vi "Post-Build Action - PPL.vi"(5 "Files Generated by Build":path[](array[path]), 6 "Top Level/Always Included VIs":path[](array[path]), 7 "Destination Path":path, 8 "error in (no error)":errorcluster, 9 "Target Name":string, 10 "Build Specification Name":string, 11 "Project Path":path) -> (0 "error out":errorcluster)   [LabVIEW 2020]
doc: "<b>Post-Build Action</b>\nThis vi completes any post build actions needed for properly building the plugin."
uses:
  <vilib>/ADAS Record/Utilities/Config/Data Converter/Data Container and Version to JSON.vi
  <vilib>/ADAS Record/Utilities/ADAS Utilities.lvlib
  PE/ADAS PE Template.lvclass
  Controller/PE Controller.lvclass
panel:
  # "#via_ignore"
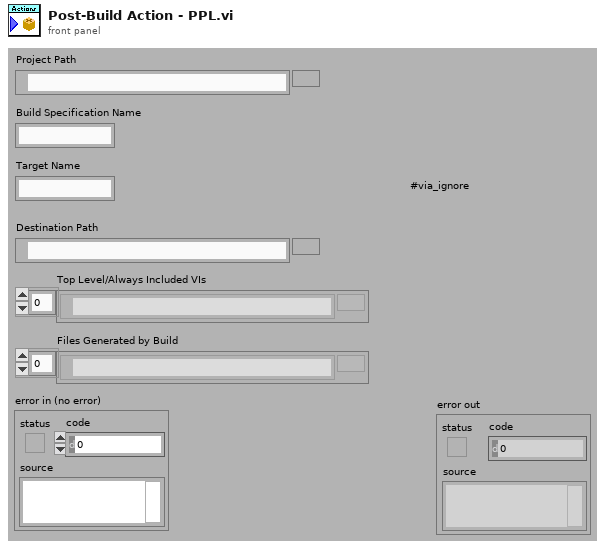
[diagram p1: front panel]
types:
  T1 = typedef "ADAS PE Template.lvlib/ADAS PE Template.lvclass/Configuration.ctl" = cluster{"Parameter1":string}
  T2 = typedef "ADAS Utilities.lvlib/Config Version.ctl" = cluster{"Major":u32, "Minor":u32, "Fix":u32, "Build":u32}
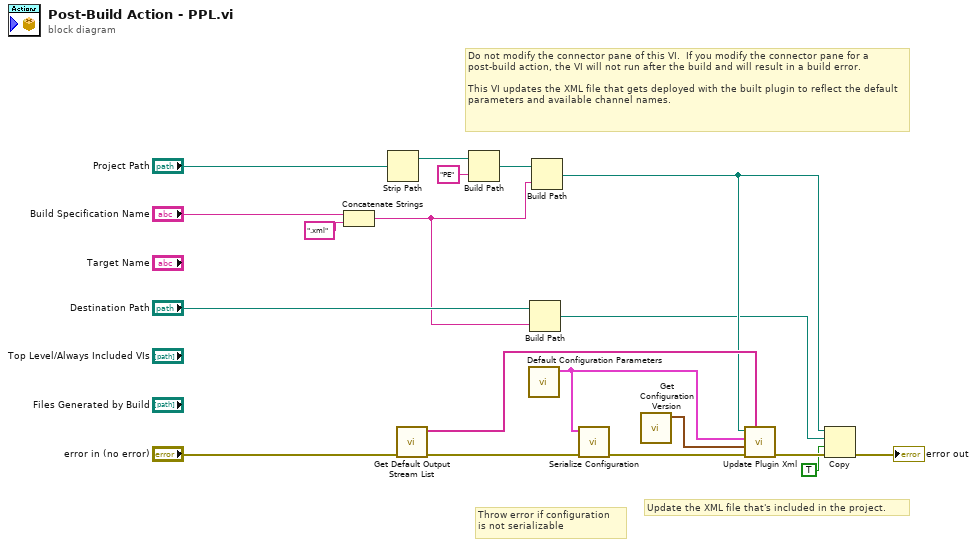
[diagram p0: block diagram]
diagram:
  # "Throw error if configuration\nis not serializable"
  # "Update the XML file that's included in the project."
  # "Do not modify the connector pane of this VI.  If you modify the connector pane for a post-build action, the VI will not run after the build and will result in a build error.\n\nThis VI updates the XML file that gets deployed with the built plugin to reflect the default parameters and available channel names."
  n1 = Concatenate Strings("Build Specification Name", ".xml" ("string")) -> (w3:string)
  n2 = Strip Path(path="Project Path") -> (stripped path=w18:path)  [unwired: 1 out]
  n3 = call "Get Default Output Stream List.vi"("error in (no error)"="error in (no error)") -> ("error out"=w10:errorcluster, "Output Streams"=w9:string[])  [unwired: 9 in]
  n4 = Build Path(base path=w18, name or relative path="PE") -> (appended path=w16:path)
  n5 = call "Default Configuration Parameters.vi"() -> ("Default Configuration"=w1:T1)  [unwired: 11 in]
  n6 = Build Path(base path="Destination Path", name or relative path=w3) -> (appended path=w5:path)
  n7 = Build Path(base path=w16, name or relative path=w3) -> (appended path=w7:path)
  n8 = call "Serialize Configuration.vi"("error in (no error)"=w10, "Configuration"=w1) -> ("error out"=w2:errorcluster)  [unwired: 8 in, 1 out]
  n9 = call "Get Configuration Version.vi"() -> ("Version"=w12:T2)  [unwired: 11 in]
  n10 = call <vilib>:"Update Plugin Xml.vi"("Output Channels"=w9, "error in (no error)"=w2, "Version"=w12, "Plugin Config"=w1, "XML Path"=w7) -> ("error out"=w13:errorcluster)  [unwired: 6 in]
  n11 = Copy(8:w13, 9:TRUE ("overwrite (F)"), 10:w5, 11:w7) -> (0:→"error out":errorcluster)  [unwired: 1 in, 2 out]
